vi "Add Event.vi"(8 "error in (no error)":errorcluster, 10 "Event Name":string="acquireFixation", 11 "TCP Network Connection Refnum":refnum<k5>) -> (0 "error out":errorcluster, 3 "connection ID out":refnum<k5>)   [LabVIEW 2010]
uses:
  Matlab API.lvlib
  Core SubVIs/Core SubVIs.lvlib
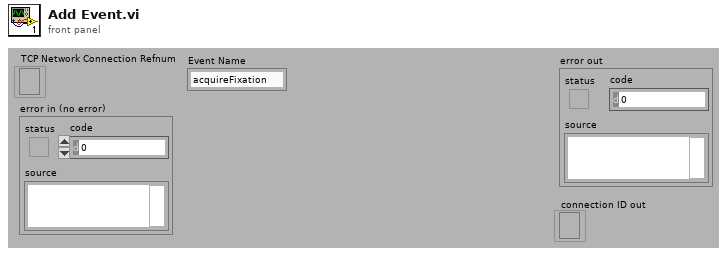
[diagram p1: front panel]
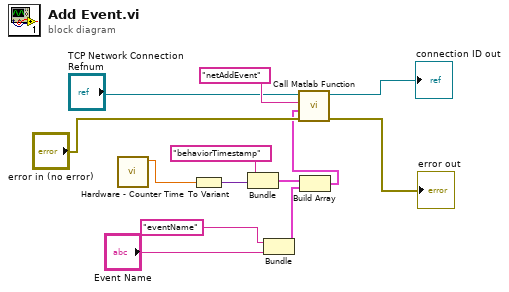
[diagram p0: block diagram]
diagram:
  n1 = call "Hardware - Counter Time.vi"() -> ("Timer Value (ms)"=w2:dbl)  [unwired: 10 in, 1 out]
  n2 = To Variant(anything=w2) -> (Variant=w3:variant)
  n3 = Bundle("behaviorTimestamp", "Variant"=w3) -> (w11:cluster{string, "Variant":variant})  [unwired: 1 in]
  n4 = Bundle("eventName", "Event Name"="Event Name") -> (w9:cluster{string, "Event Name":string})  [unwired: 1 in]
  n5 = Build Array(w11, w9) -> (w1:cluster{string, "Variant":variant}[])
  n6 = call "Call Matlab Function.vi"("error in (no error)"="error in (no error)", "Matlab Param Array"=w1, "Function name"="netAddEvent", "TCP Network Connection Refnum"="TCP Network Connection Refnum") -> ("error out"=→"error out":errorcluster, "connection ID out"=→"connection ID out":refnum<k5>)  [unwired: 4 in, 2 out]
